vi "new.vi"(8 "error in (no error)":errorcluster, 11 "IDoublyNode in":refnum<class "IDoublyNode.lvclass">) -> (0 "error out":errorcluster, 3 "node ref":refnum<data-value>)   [LabVIEW 2021, in "IDoublyNode.lvclass"]
uses:
  IDoublyNode.lvclass
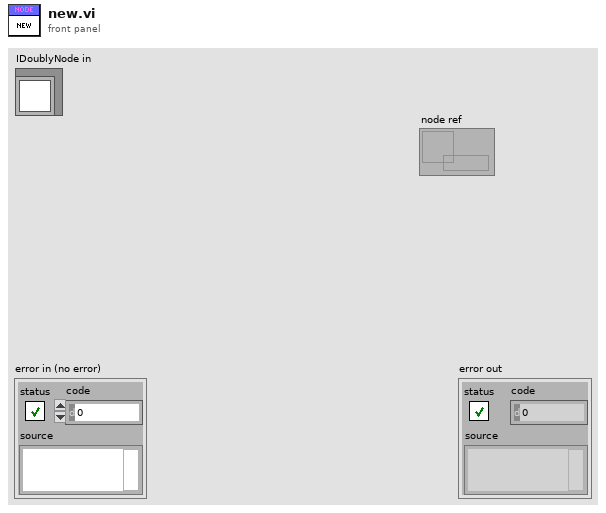
[diagram p1: front panel]
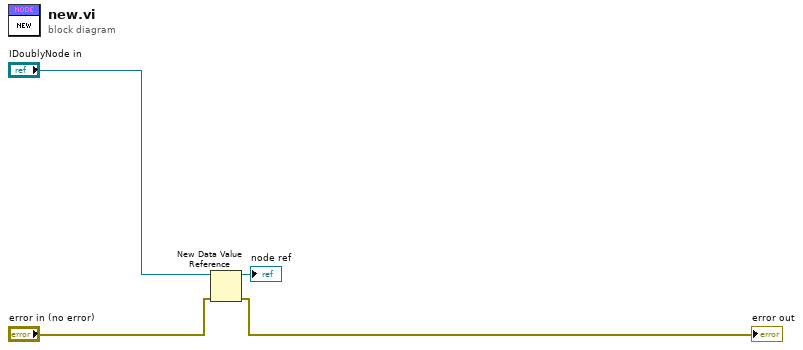
[diagram p0: block diagram]
diagram:
  n1 = New Data Value Reference(data value="IDoublyNode in", error in="error in (no error)") -> (data value reference=→"node ref":refnum<data-value>, error out=→"error out":errorcluster)
